vi "Power Array to Cluster.vi"(11 "Output Power Data":sgl[](array[numeric])) -> (3 "PowerData 2":T1 {"Lambda:Element 2" format="%.3g"; "Lambda:Element 1" format="%.3g"; "S:Element 2" format="%.3g"; "S:Element 1" format="%.3g"; "Freq U:Element 1" format="%.3g"; "Time:Element 1" format="%.3g"; "Cf U:Element 2" format="%.3g"; "Cf U:Element 1" format="%.3g"; "Uthd:Element 2" format="%.3g"; "Uthd:Element 1" format="%.3g"; "Cf I:Element 2" format="%.3g"; "Cf I:Element 1" format="%.3g"; "Urms:Element 1" format="%.3g"; "Urms:Element 2" format="%.3g"; "Wp:Sigma" format="%.3g"; "P:Sigma" format="%.3g"; "Irms:Element 2" format="%.3g"; "Irms:Element 1" format="%.3g"})   [LabVIEW 2013]
uses:
  Utility/Standby Power/Type Definitions/Power Data.ctl
panel:
  in  "PowerData":T1 {"Lambda:Element 2" format="%.3g"; "Lambda:Element 1" format="%.3g"; "S:Element 2" format="%.3g"; "S:Element 1" format="%.3g"; "Freq U:Element 1" format="%.3g"; "Time:Element 1" format="%.3g"; "Cf U:Element 2" format="%.3g"; "Cf U:Element 1" format="%.3g"; "Uthd:Element 2" format="%.3g"; "Uthd:Element 1" format="%.3g"; "Cf I:Element 2" format="%.3g"; "Cf I:Element 1" format="%.3g"; "Urms:Element 1" format="%.3g"; "Urms:Element 2" format="%.3g"; "Wp:Sigma" format="%.3g"; "P:Sigma" format="%.3g"; "Irms:Element 2" format="%.3g"; "Irms:Element 1" format="%.3g"}
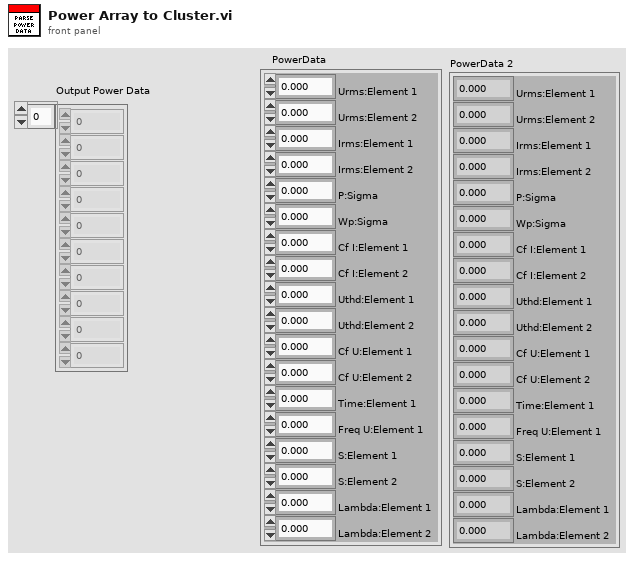
[diagram p1: front panel]
types:
  T1 = typedef "Power Data.ctl" = cluster{"Irms:Element 1":dbl, "Irms:Element 2":dbl, "P:Sigma":dbl, "Wp:Sigma":dbl, "Urms:Element 2":dbl, "Urms:Element 1":dbl, "Cf I:Element 1":dbl, "Cf I:Element 2":dbl, "Uthd:Element 1":dbl, "Uthd:Element 2":dbl, "Cf U:Element 1":dbl, "Cf U:Element 2":dbl, "Time:Element 1":dbl, "Freq U:Element 1":dbl, "S:Element 1":dbl, "S:Element 2":dbl, "Lambda:Element 1":dbl, "Lambda:Element 2":dbl}
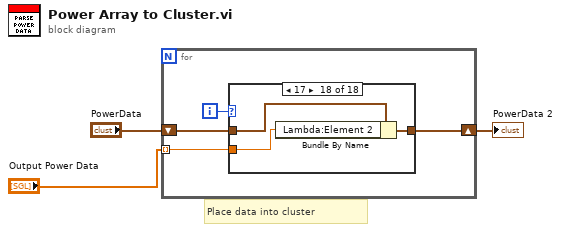
[diagram p0: block diagram]
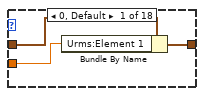
[diagram p2: hidden frame]
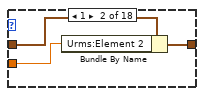
[diagram p3: hidden frame]
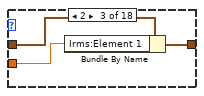
[diagram p4: hidden frame]
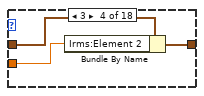
[diagram p5: hidden frame]
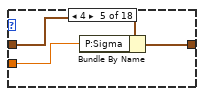
[diagram p6: hidden frame]
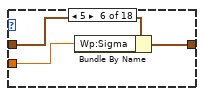
[diagram p7: hidden frame]
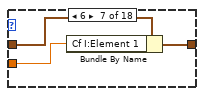
[diagram p8: hidden frame]
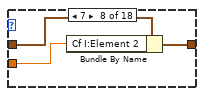
[diagram p9: hidden frame]
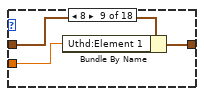
[diagram p10: hidden frame]
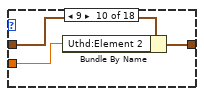
[diagram p11: hidden frame]
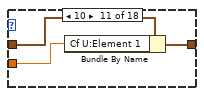
[diagram p12: hidden frame]
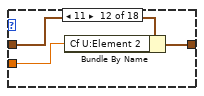
[diagram p13: hidden frame]
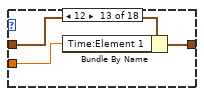
[diagram p14: hidden frame]
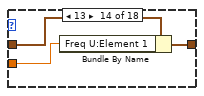
[diagram p15: hidden frame]
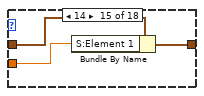
[diagram p16: hidden frame]
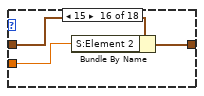
[diagram p17: hidden frame]
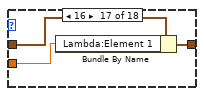
[diagram p18: hidden frame]
diagram:
  # "Place data into cluster"
  n1 = for {
    tunnel: "Output Power Data" -> [w6] mode=indexing
    shift-right: [w4] -> w1
    shift-left: "PowerData" -> [w5]
    i -> [w7]
    n2 = case shown="17" w7 {
      tunnel: w6 -> [w10 w13 w16 w19 w22 w25 w28 w31 w34 w36 w38 w41 w44 w47 w50 w53 w56 w59]
      tunnel: [w9 w12 w15 w18 w21 w24 w27 w30 w33 w37 w39 w42 w45 w48 w51 w54 w57 w60] -> w4
      tunnel: w5 -> [w8 w11 w14 w17 w20 w23 w26 w29 w32 w35 w40 w43 w46 w49 w52 w55 w58 w61]
      frame 0, Default {
        n3 = Bundle By Name(cluster=w8, "Urms:Element 1"=w10) -> (w9:T1)
      }
      frame 1 {
        n4 = Bundle By Name(cluster=w11, "Urms:Element 2"=w13) -> (w12:T1)
      }
      frame 2 {
        n5 = Bundle By Name(cluster=w14, "Irms:Element 1"=w16) -> (w15:T1)
      }
      frame 3 {
        n6 = Bundle By Name(cluster=w17, "Irms:Element 2"=w19) -> (w18:T1)
      }
      frame 4 {
        n7 = Bundle By Name(cluster=w20, "P:Sigma"=w22) -> (w21:T1)
      }
      frame 5 {
        n8 = Bundle By Name(cluster=w23, "Wp:Sigma"=w25) -> (w24:T1)
      }
      frame 6 {
        n9 = Bundle By Name(cluster=w26, "Cf I:Element 1"=w28) -> (w27:T1)
      }
      frame 7 {
        n10 = Bundle By Name(cluster=w29, "Cf I:Element 2"=w31) -> (w30:T1)
      }
      frame 8 {
        n11 = Bundle By Name(cluster=w32, "Uthd:Element 1"=w34) -> (w33:T1)
      }
      frame 9 {
        n12 = Bundle By Name(cluster=w35, "Uthd:Element 2"=w36) -> (w37:T1)
      }
      frame 10 {
        n13 = Bundle By Name(cluster=w40, "Cf U:Element 1"=w38) -> (w39:T1)
      }
      frame 11 {
        n14 = Bundle By Name(cluster=w43, "Cf U:Element 2"=w41) -> (w42:T1)
      }
      frame 12 {
        n15 = Bundle By Name(cluster=w46, "Time:Element 1"=w44) -> (w45:T1)
      }
      frame 13 {
        n16 = Bundle By Name(cluster=w49, "Freq U:Element 1"=w47) -> (w48:T1)
      }
      frame 14 {
        n17 = Bundle By Name(cluster=w52, "S:Element 1"=w50) -> (w51:T1)
      }
      frame 15 {
        n18 = Bundle By Name(cluster=w55, "S:Element 2"=w53) -> (w54:T1)
      }
      frame 16 {
        n19 = Bundle By Name(cluster=w58, "Lambda:Element 1"=w56) -> (w57:T1)
      }
      frame 17 {
        n20 = Bundle By Name(cluster=w61, "Lambda:Element 2"=w59) -> (w60:T1)
      }
    }
  }
  "PowerData 2" <- w1
